vi "Read ref.vi"(8 "error in (no error)":errorcluster, 11 "stats in":refnum<class "stats.lvclass">) -> (0 "error out":errorcluster, 2 "ref":refnum<vi>, 3 "stats out":refnum<class "stats.lvclass">)   [LabVIEW 2016, in "stats.lvclass"]
uses:
  stats.lvclass
  stats.lvclass/stats.ctl
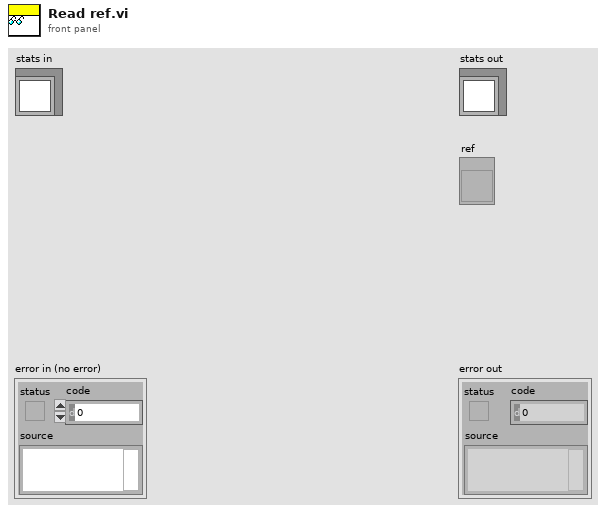
[diagram p1: front panel]
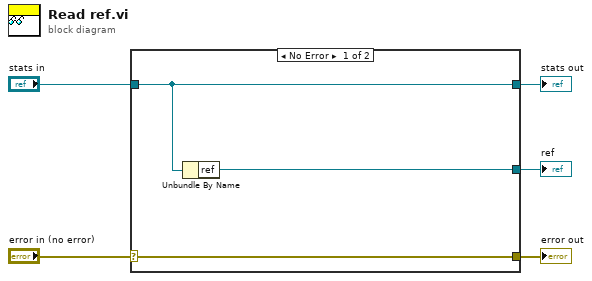
[diagram p0: block diagram]
diagram:
  n1 = case shown="No Error" "error in (no error)" {
    selector: "error in (no error)" -> [w8 w9]
    tunnel: [w8 w9] -> w4
    tunnel: [w7 w10] -> w2
    tunnel: "stats in" -> [w7 w10]
    tunnel: [w6 _] -> w1
    frame No Error {
      n2 = Unbundle By Name(w7) -> ("ref"=w6:refnum<vi>)
    }
    frame Error {
    }
  }
  "error out" <- w4
  "stats out" <- w2
  "ref" <- w1
